vi "main_auto_cleanup.vi"(10 "Cleanup?":refnum<vi>) -> ()   [LabVIEW 2019]
uses:
  lib/libSimulationControl/libSimulationControl.lvlib
panel:
  # "*******************************************************************\nBiogas Plant Control\n\nAuthor: Paul Zügel\nGCSC-Frankfurt am Main 2020\n\n*******************************************************************"
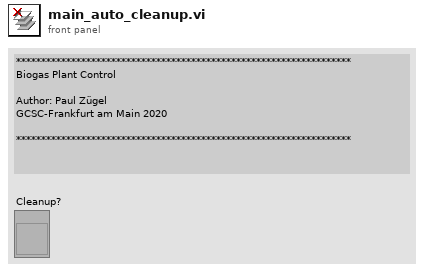
[diagram p1: front panel]
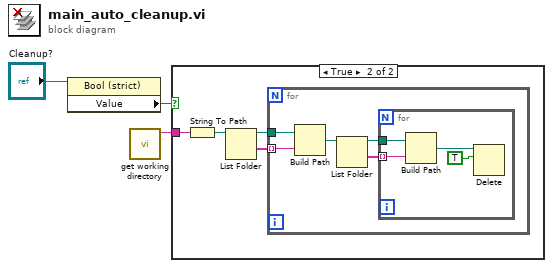
[diagram p0: block diagram]
diagram:
  # "Delete all subfolders"
  n1 = property on="Property Node" class="Bool (strict)"(reference="Cleanup?") -> ("Value"=w1:bool)  [unwired: 1 in, 2 out]
  n2 = call "get working directory.vi"() -> ("function return"=w3:string)  [unwired: 10 in, 1 out]
  n3 = case shown="True" w1 {
    tunnel: w3 -> [_ w4]
    frame False {
    }
    frame True {
      n4 = String To Path(string=w4) -> (path=w6:path)
      n5 = List Folder(path=w6) -> (path out=w5:path, folder names=w7:string[])  [unwired: 3 in, 2 out]
      n6 = for {
        tunnel: w7 -> [w11] mode=indexing
        tunnel: w5 -> [w12]
        n7 = Build Path(base path=w12, name or relative path=w11) -> (appended path=w10:path)
        n8 = List Folder(path=w10) -> (path out=w8:path, folder names=w9:string[])  [unwired: 3 in, 2 out]
        n9 = for {
          tunnel: w9 -> [w15] mode=indexing
          tunnel: w8 -> [w16]
          n10 = Build Path(base path=w16, name or relative path=w15) -> (appended path=w14:path)
          n11 = Delete(path (use dialog)=w14, entire hierarchy (F)=TRUE) -> ()  [unwired: 3 in, 3 out]
        }
      }
    }
  }
